vi "Test Escape String for Windows.vi"() -> (0 "error out":errorcluster)   [LabVIEW 2025]
doc: "Validates that a single argument string is correctly escaped according to Windows command-line rules when quoting is required. The test verifies proper handling of quotes, backslashes before quotes, and trailing backslashes to ensure the argument is interpreted correctly by the target process."
uses:
  <vilib>/addons/_JKI Toolkits/Caraya/classes/Test/Test.lvclass
  src/Process Executor/Process Executor.lvclass
  <vilib>/addons/_JKI Toolkits/Caraya/classes/Assert/Assert.lvclass
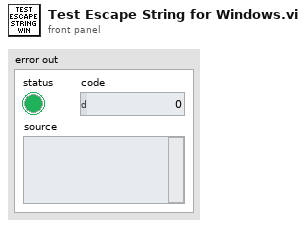
[diagram p1: front panel]
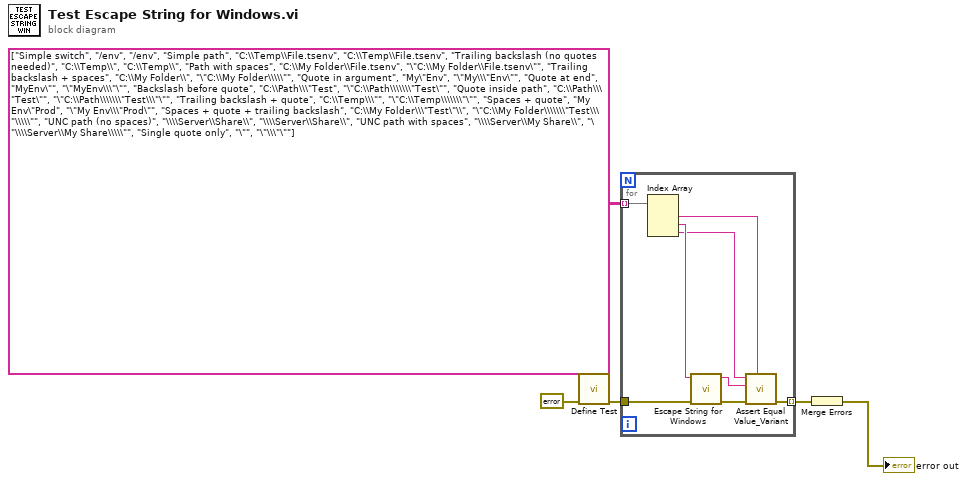
[diagram p0: block diagram]
diagram:
  n1 = call <vilib>:"Define Test.vi"("error in (no error)"=errorcluster {"status"=FALSE, "code"=0, "source"=""}) -> ("error out"=w4:errorcluster)  [unwired: 9 in, 1 out]
  n2 = for {
    tunnel: w4 -> [w11]
    tunnel: string[][] [["Simple switch", "/env", "/env"], ["Simple path", "C:\\Temp\\File.tsenv", "C:\\Temp\\File.tsenv"], ["Trailing backslash (no quotes needed)", "C:\\Temp\\", "C:\\Temp\\"], ["Path with spaces", "C:\\My Folder\\File.tsenv", "\"C:\\My Folder\\File.tsenv\""], ["Trailing backslash + spaces", "C:\\My Folder\\", "\"C:\\My Folder\\\\\""], ["Quote in argument", "My\"Env", "\"My\\\"Env\""], ["Quote at end", "MyEnv\"", "\"MyEnv\\\"\""], ["Backslash before quote", "C:\\Path\\\"Test", "\"C:\\Path\\\\\\\"Test\""], ["Quote inside path", "C:\\Path\\\"Test\"", "\"C:\\Path\\\\\\\"Test\\\"\""], ["Trailing backslash + quote", "C:\\Temp\\\"", "\"C:\\Temp\\\\\\\"\""], ["Spaces + quote", "My Env\"Prod", "\"My Env\\\"Prod\""], ["Spaces + quote + trailing backslash", "C:\\My Folder\\\"Test\"\\", "\"C:\\My Folder\\\\\\\"Test\\\"\\\\\""], ["UNC path (no spaces)", "\\\\Server\\Share\\", "\\\\Server\\Share\\"], ["UNC path with spaces", "\\\\Server\\My Share\\", "\"\\\\Server\\My Share\\\\\""], ["Single quote only", "\"", "\"\\\"\""]] -> [w10] mode=indexing
    tunnel: [w6] -> w1 mode=indexing
    n3 = Index Array(array=w10) -> (element #1=w9:string, element #2=w8:string, element #3=w7:string)  [unwired: 3 in]
    n4 = call "Escape String for Windows.vi"("error in"=w11, "String in"=w8) -> ("error out"=w12:errorcluster, "String out"=w13:string)  [unwired: 8 in]
    n5 = call <vilib>:"Assert Equal Value_Variant.vi"("Label"=w9, "error in (no error)"=w12, "Actual"=w13, "Expected"=w7) -> ("error out"=w6:errorcluster)  [unwired: 6 in, 1 out]
  }
  n6 = Merge Errors(w1) -> (→"error out":errorcluster)
